vi "Initialize Front Panel.vi"(8 "error in (no error)":errorcluster, 11 "BoundViewManager in":refnum<class "BoundViewManager.lvclass">) -> (0 "error out":errorcluster, 3 "BoundViewManager out":refnum<class "BoundViewManager.lvclass">)   [LabVIEW 2018, in "MVA Framework.lvlib" / "BoundViewManager.lvlib" / "BoundViewManager.lvclass"]
doc: "初始化前面板"
uses:
  BoundViewManager.lvclass
  <vilib>/ActorFramework/Message Enqueuer/Message Enqueuer.lvclass
  modules/mva-viewable/Source/IViewable/IViewable Messages/Insert Front Panel Msg/Insert Front Panel Msg.lvclass
  61cc6e39-6280-4a2f-9646-d72848929907.vi
  modules/mva-viewable/Source/IViewManager/IViewManager/IViewManager.lvclass
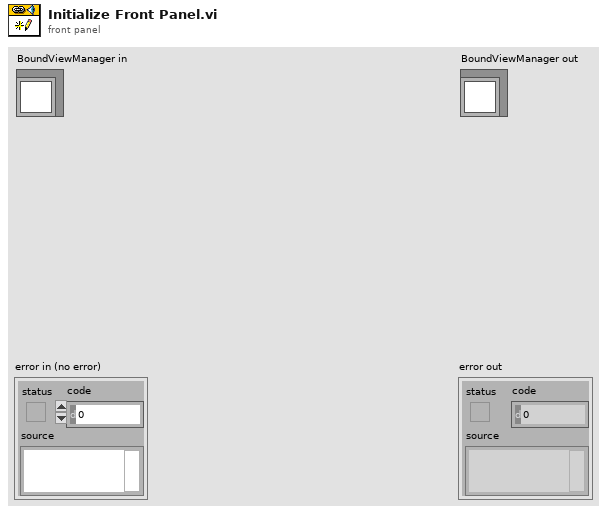
[diagram p1: front panel]
types:
  T1 = typedef "MVA Framework.lvlib/IViewable.lvlib/ProtectedSubpanel.lvclass/Protected Subpanel Reference.ctl" = refnum<data-value>
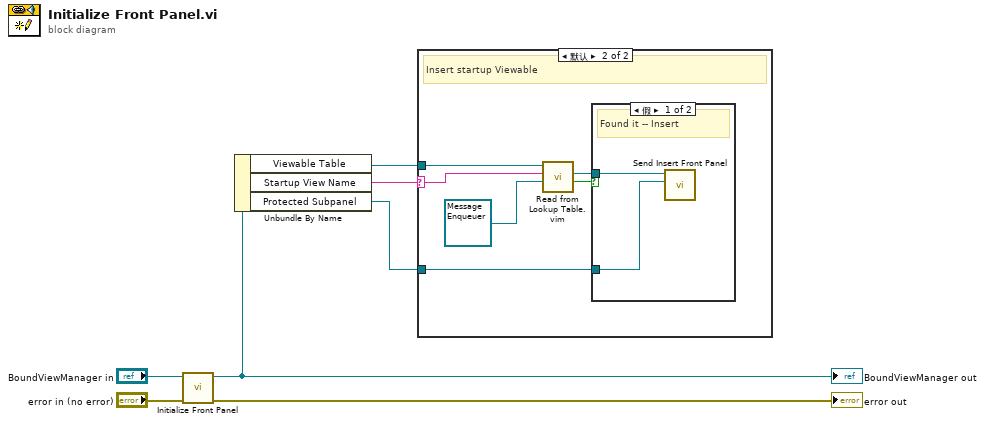
[diagram p0: block diagram]
diagram:
  n1 = call-parent "Initialize Front Panel.vi"("error in (no error)"="error in (no error)", "IViewable in"="BoundViewManager in") -> ("error out"=→"error out":errorcluster, "IViewable out"=w4:refnum<class "BoundViewManager.lvclass">)  [unwired: 8 in]
  "BoundViewManager out" <- w4
  n2 = Unbundle By Name(w4) -> ("Viewable Table"=w2:refnum<data-value>, "Startup View Name"=w3:string, "Protected Subpanel"=w1:T1)
  n3 = case shown="默认" w3 {
    selector: w3 -> [_ w12]
    tunnel: w2 -> [_ w13]
    tunnel: w1 -> [_ w9]
    frame "" {
      # "No startup viewable insertion"
    }
    frame Default {
      # "Insert startup Viewable"
      n4 = call "Read from Lookup Table.vim"("Type"=refnum<class "Message Enqueuer.lvclass"> refnum ("Message Enqueuer"), "Item Name"=w12, "LookupTable Reference"=w13) -> ("Not Found?"=w11:bool, "Value"=w10:refnum<class "Message Enqueuer.lvclass">)  [unwired: 5 in, 2 out]
      n5 = case shown="假" w11 {
        tunnel: w10 -> [w14 _]
        tunnel: w9 -> [w15 _]
        frame False {
          # "Found it -- Insert"
          n6 = call "Send Insert Front Panel.vi"("Protected Subpanel"=w15, "Message Enqueuer"=w14) -> ()  [unwired: 8 in, 2 out]
        }
        frame True {
          # "Not found"
        }
      }
    }
  }
